vi "ROI grp-Window-New POI group name.vi"() -> (1 "Group Name out":string, 3 "Cancelled?":bool)   [LabVIEW 2017]
uses:
  <vilib>/Utility/miscctls.llb/LVPointTypeDef.ctl
  Typedefs/Get-Set-Clear Control.ctl
panel:
  in  "Cancel":bool
  in  "Group Name":string caption="Enter a name for the new group"
  in  "OK":bool
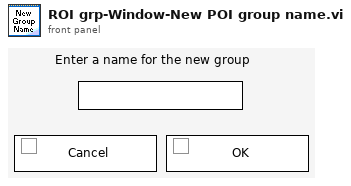
[diagram p1: front panel]
types:
  T1 = typedef "Get-Set-Clear Control.ctl" = enum16{"Get", "Set", "Clear"}
  T2 = typedef "LVPointTypeDef.ctl" = cluster{"Horizontal":i16, "Vertical":i16}
  T3 = typedef "ROI group info cluster.ctl" = cluster{"Group name":string, "# ROI in group":i32, "ROI numbers in group":i32[], "Group region specifier cluster":T4}
  T4 = typedef "ROI Descriptor" = cluster{"Global Rectangle":i32[], "Contours":cluster{"ID":enum32{"External", "Internal"}, "Type":u32, "Coordinates":i32[]}[]}
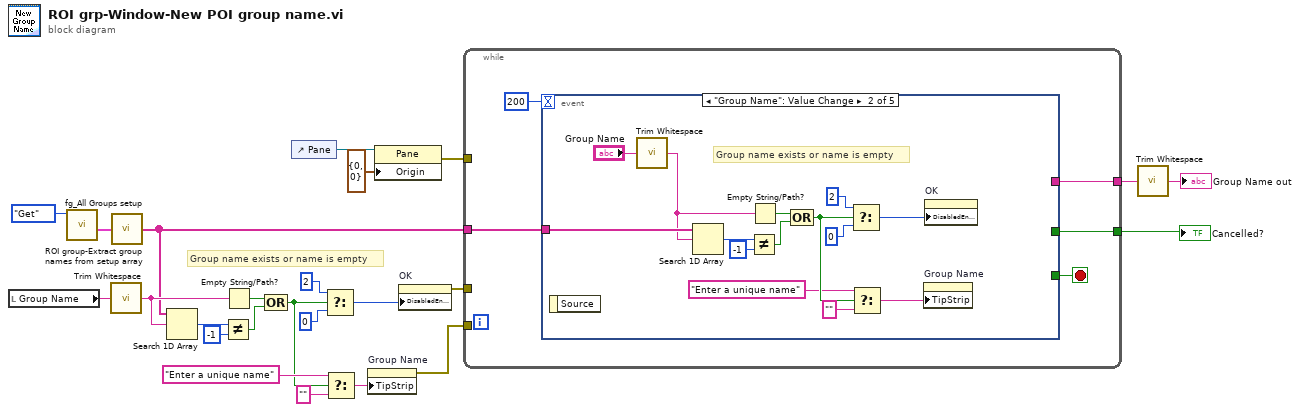
[diagram p0: block diagram]
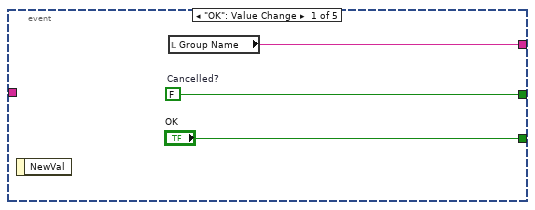
[diagram p2: hidden frame]
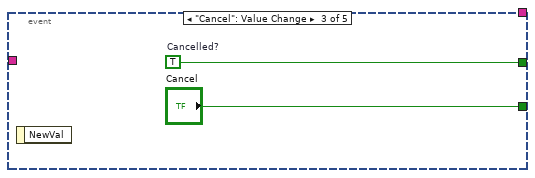
[diagram p3: hidden frame]
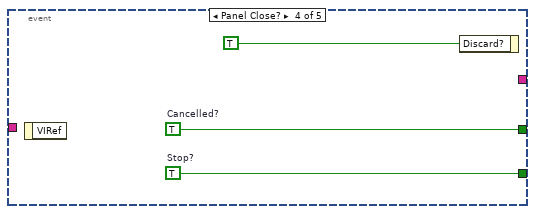
[diagram p4: hidden frame]
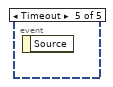
[diagram p5: hidden frame]
diagram:
  # "Group name exists or name is empty"
  n1 = local read "Group Name"() -> (w6:string)
  n2 = call "fg_All Groups setup.vi"("Function"=Get-Set-Clear_Control."Get") -> ("Groups setup out"=w20:T3[])  [unwired: 9 in, 1 out]
  n3 = call <vilib>:"Trim Whitespace.vi"("string"=w6) -> ("trimmed string"=w14:string)  [unwired: 1 in]
  n4 = call "ROI group-Extract group names from setup array.vi"("Groups setup"=w20) -> ("Group Names Array"=w4:string[])
  n5 = Search 1D Array(1D array=w4, element=w14) -> (index of element=w7:i32)  [unwired: 1 in]
  n6 = Not Equal?(x=w7, y=-1) -> (x != y?=w10:bool)
  n7 = Empty String/Path?(string/path=w14) -> (empty?=w9:bool)
  n8 = Compound Arithmetic op=OR(w9, w10) -> (w15:bool)
  n9 = control-ref of="Pane"() -> (w1:refnum<vi>)
  n10 = Select(t=2, s=w15, f=0) -> (s? t:f=w13:i32)
  n11 = Select(t="Enter a unique name" ("Tip Strip"), s=w15, f="") -> (s? t:f=w3:string)
  n12 = property on="Group Name" class="Str"("TipStrip"=w3) -> (error out=w2:errorcluster)  [unwired: 2 in, 1 out]
  n13 = property class="Pane"(reference=w1, "Origin"=T2 {"Horizontal"=0, "Vertical"=0}) -> (error out=w22:errorcluster)  [unwired: 1 in, 1 out]
  n14 = property on="OK" class="Bool"("DisabledEnum"=w13) -> (error out=w5:errorcluster)  [unwired: 2 in, 1 out]
  n15 = while {
    tunnel: [w28] -> w24
    tunnel: [w26] -> w18
    tunnel: w22 -> [_]
    tunnel: w4 -> [w25]
    tunnel: w5 -> [_]
    tunnel: w2 -> [_]
    stop <- w29 stop-if-true
    n16 = event shown="[1] \"Group Name\": Value Change" {
      selector: _ -> [_ _ _ _ _]
      dyn-events: _ -> [_ _ _ _ _]
      timeout: 200 -> [_ _ _ _ _]
      tunnel: ["OK" _ "Cancel" w50 _] -> w29
      tunnel: [w32 _ w48 w49 _] -> w28
      tunnel: [w30 _ _ _ _] -> w26
      tunnel: w25 -> [_ w46 _ _ _]
      event "OK": Value Change {
        w32 = FALSE  # Cancelled?
        n17 = event-data() -> ()  [unwired: 1 in, 1 out]
        n18 = local read "Group Name"() -> (w30:string)
      }
      event "Group Name": Value Change {
        # "Group name exists or name is empty"
        n19 = event-data() -> ()  [unwired: 1 in, 1 out]
        n20 = call <vilib>:"Trim Whitespace.vi"("string"="Group Name") -> ("trimmed string"=w37:string)  [unwired: 1 in]
        n21 = Search 1D Array(1D array=w46, element=w37) -> (index of element=w45:i32)  [unwired: 1 in]
        n22 = Not Equal?(x=w45, y=-1) -> (x != y?=w41:bool)
        n23 = Empty String/Path?(string/path=w37) -> (empty?=w42:bool)
        n24 = Compound Arithmetic op=OR(w42, w41) -> (w36:bool)
        n25 = Select(t=2, s=w36, f=0) -> (s? t:f=w38:i32)
        n26 = Select(t="Enter a unique name" ("Tip Strip"), s=w36, f="") -> (s? t:f=w34:string)
        n27 = property on="Group Name" class="Str"("TipStrip"=w34) -> ()  [unwired: 2 in, 2 out]
        n28 = property on="OK" class="Bool"("DisabledEnum"=w38) -> ()  [unwired: 2 in, 2 out]
      }
      event "Cancel": Value Change {
        w48 = TRUE  # Cancelled?
        n29 = event-data() -> ()  [unwired: 1 in, 1 out]
      }
      event Panel Close? {
        w49 = TRUE  # Cancelled?
        w50 = TRUE  # Stop?
        n30 = event-data() -> ()  [unwired: 1 in, 1 out]
        n31 = event-data("Discard?"=TRUE) -> ()  [unwired: 1 in, 1 out]
      }
      event Timeout {
        n32 = event-data() -> ()  [unwired: 1 in, 1 out]
      }
    }
  }
  "Cancelled?" <- w24
  n33 = call <vilib>:"Trim Whitespace.vi"("string"=w18) -> ("trimmed string"=→"Group Name out":string)  [unwired: 1 in]
